vi "Get Data.vi"(8 "error in (no error)":errorcluster, 10 "Bus In":refnum<class "Bus.lvclass">, 11 "Single Query in":refnum<class "Multiple Queries.lvclass">) -> (0 "error out":errorcluster, 1 "String Read":string, 2 "Bus Out":refnum<class "Bus.lvclass">, 3 "Single Query out":refnum<class "Multiple Queries.lvclass">)   [LabVIEW 2018, in "Multiple Queries.lvclass"]
doc: "Single Query.lvclass:Get Data.vi\n\nThis VI does a Query and a Response for the Single Query instance of the Query class.\n\nInstrument Communication Module Version 1.0\nDecember, 2017 Original Code Consulting David Thomson\n www.originalcode.com"
uses:
  Multiple Queries.lvclass
  Bus/Bus.lvclass
  Multiple Queries.lvclass/Multiple Queries.ctl
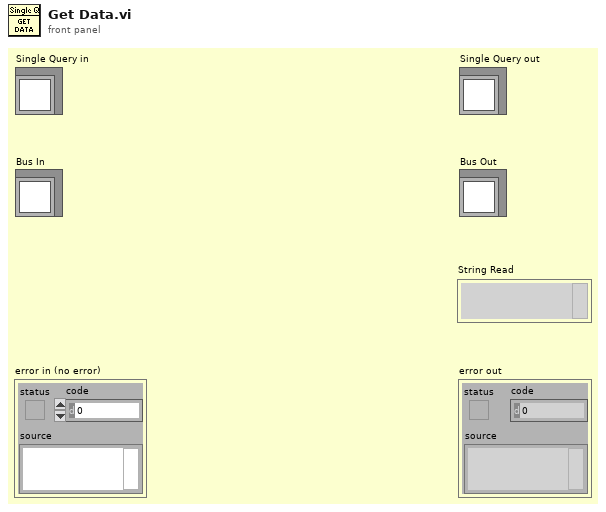
[diagram p1: front panel]
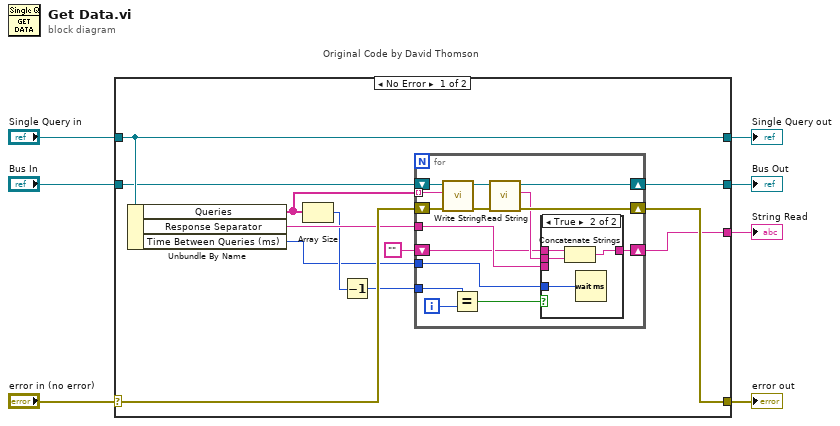
[diagram p0: block diagram]
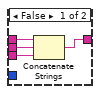
[diagram p2: hidden frame]
diagram:
  n1 = case "Original Code by David Thomson" shown="No Error" "error in (no error)" {
    selector: "error in (no error)" -> [w15 w45]
    tunnel: [w18 w45] -> w6
    tunnel: [w17 w44] -> w4
    tunnel: "Single Query in" -> [w17 w44]
    tunnel: [w19 w43] -> w3
    tunnel: "Bus In" -> [w16 w43]
    tunnel: [w12 _] -> w1
    frame No Error {
      n2 = Unbundle By Name(w17) -> ("Queries"=w11:string[], "Response Separator"=w13:string, "Time Between Queries (ms)"=w8:u32)
      n3 = Array Size(array=w11) -> (size(s)=w10:i32)
      n4 = Decrement(x=w10) -> (x-1=w9:i32)
      n5 = for {
        tunnel: w11 -> [w30] mode=indexing
        shift-right: [w34] -> w19
        shift-left: w16 -> [w32]
        shift-right: [w33] -> w18
        shift-left: w15 -> [w29]
        shift-right: [w21] -> w12
        shift-left: "" -> [w22]
        tunnel: w13 -> [w23]
        tunnel: w9 -> [w26]
        tunnel: w8 -> [w20]
        i -> [w27]
        n6 = call-dynamic "Write String.vi"("error in (no error)"=w29, "String"=w30, "Bus in"=w32) -> ("error out"=w28:errorcluster, "Bus out"=w31:refnum<class "Bus.lvclass">)  [unwired: 7 in]
        n7 = Equal?(x=w26, y=w27) -> (x = y?=w25:bool)
        n8 = call-dynamic "Read String.vi"("error in (no error)"=w28, "Bus in"=w31) -> ("error out"=w33:errorcluster, "String Read"=w24:string, "Bus out"=w34:refnum<class "Bus.lvclass">)  [unwired: 6 in, 1 out]
        n9 = case shown="True" w25 {
          tunnel: w24 -> [w37 w41]
          tunnel: w23 -> [w36 _]
          tunnel: w22 -> [w38 w42]
          tunnel: [w35 w40] -> w21
          tunnel: w20 -> [_ w39]
          frame False {
            n10 = Concatenate Strings(w38, w37, w36) -> (w35:string)
          }
          frame True {
            n11 = Concatenate Strings(w42, w41) -> (w40:string)
            n12 = Wait (ms)(milliseconds to wait=w39) -> ()  [unwired: 1 out]
          }
        }
      }
    }
    frame Error {
    }
  }
  "error out" <- w6
  "Single Query out" <- w4
  "Bus Out" <- w3
  "String Read" <- w1
